vi "cic_interpolator_test_5_5cycles.vi"() -> ()   [LabVIEW 2013]
uses:
  <vilib>/measure/maspectr.llb/Power Spectrum and PSD Export Mode.ctl
  <vilib>/measure/maspectr.llb/FFT Power Spectrum and PSD for 1 Chan.vi
  <vilib>/measure/NI_MABase.lvlib
  <vilib>/measure/NI_MAPro.lvlib
panel:
  out "Waveform Graph out":dbl[](graph)
  out "Power spectrum in":cluster{"f0":dbl, "df":dbl, "magnitude":dbl[]}(graph)
  out "Power spectrum":cluster{"f0":dbl, "df":dbl, "magnitude":dbl[]}(graph)
  out "Waveform Graph":dbl[](graph)
  out "# of Iterations":i32
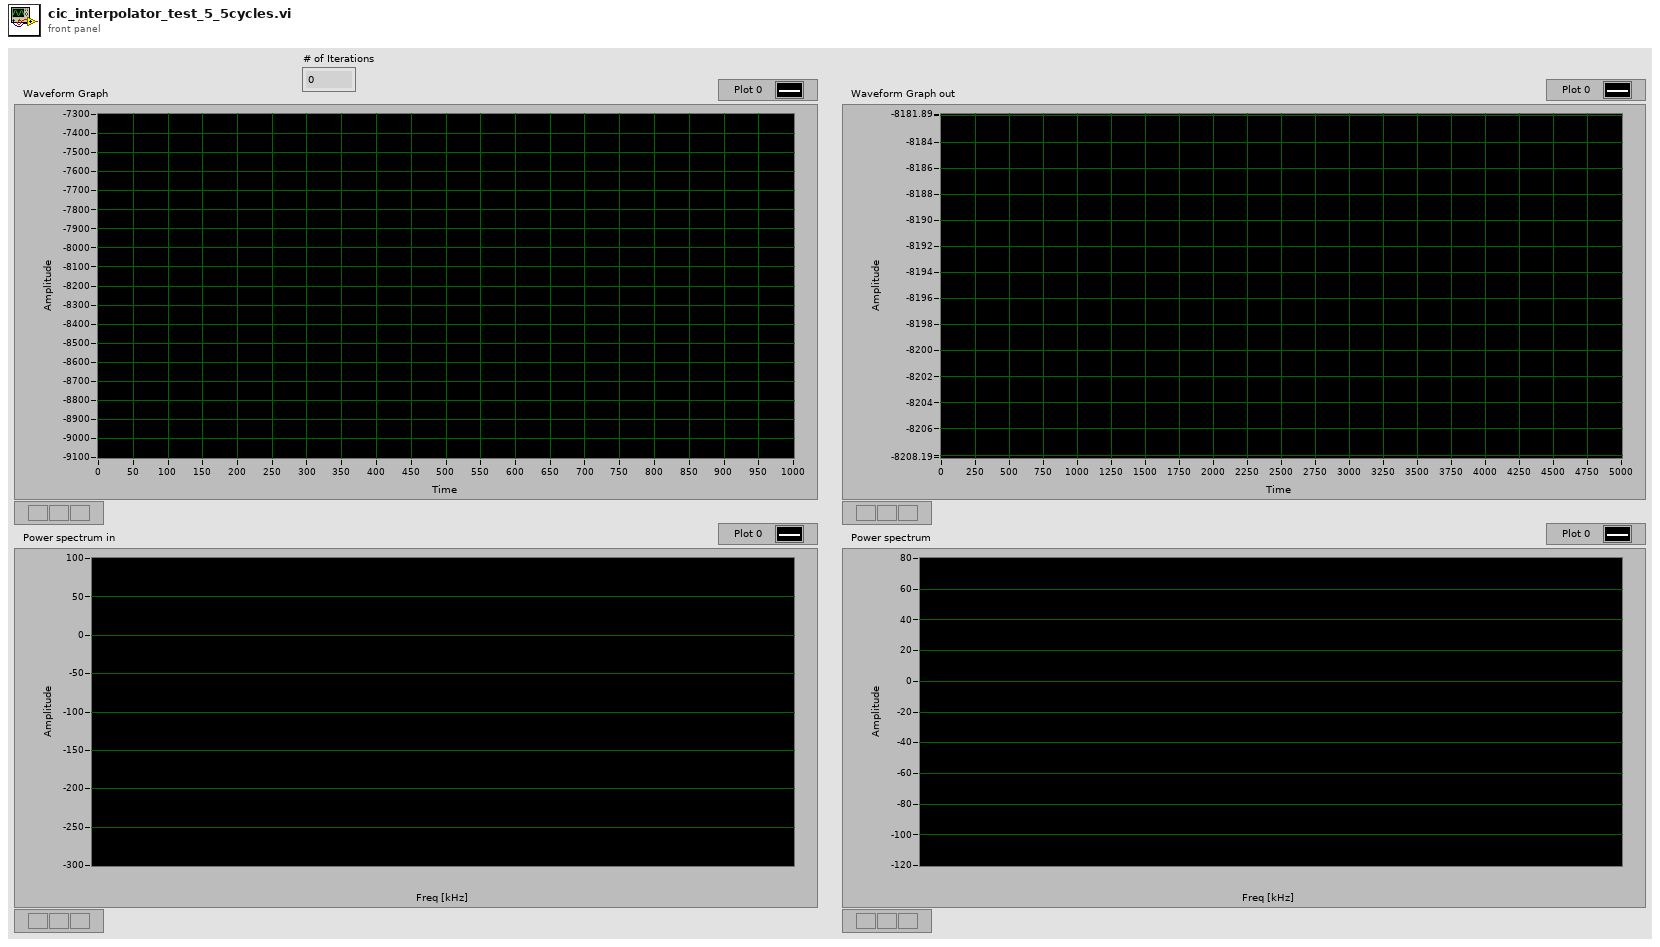
[diagram p1: front panel]
types:
  T1 = typedef "NI_MAPro.lvlib/Power Spectrum and PSD Export Mode.ctl" = u16
  T2 = cluster{"frequency":dbl, "amplitude":dbl, "phase":dbl}[]
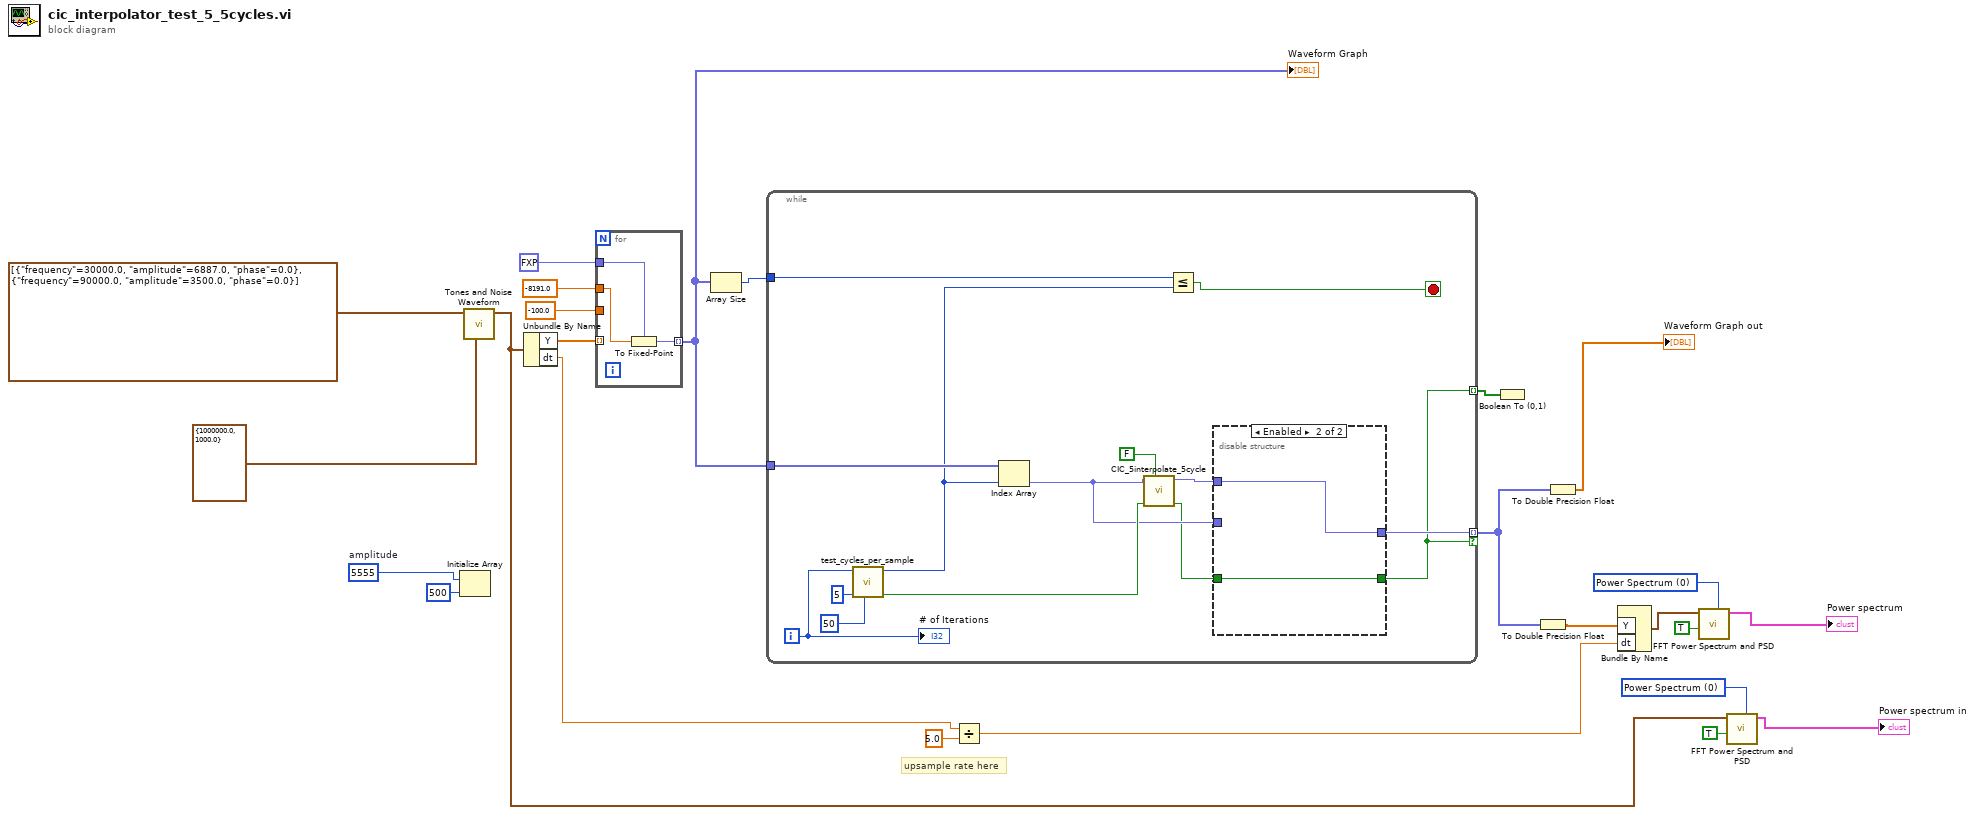
[diagram p0: block diagram]
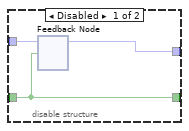
[diagram p2: hidden frame]
diagram:
  w4 = 5555  # amplitude
  w13 = T1 0 items=["Power Spectrum", "Power Spectral Density"] ("export mode")
  w21 = T1 0 items=["Power Spectrum", "Power Spectral Density"] ("export mode")
  # "upsample rate here"
  n1 = Initialize Array(w4, 500 ("dimension size")) -> ()  [unwired: 1 out]
  n2 = call <vilib>:"Tones and Noise Waveform.vi"("sampling info"=cluster{"Fs":dbl, "#s":dbl} {"Fs"=1000000.0, "#s"=1000.0}, "tones"=T2 [{"frequency"=30000.0, "amplitude"=6887.0, "phase"=0.0}, {"frequency"=90000.0, "amplitude"=3500.0, "phase"=0.0}]) -> ("signal out"=w12:waveform(dbl))  [unwired: 8 in, 1 out]
  n3 = Unbundle By Name(w12) -> ("Y"=w3:dbl[], "dt"=w19:dbl)
  n4 = for {
    tunnel: w3 -> [_] mode=indexing
    tunnel: fxp<+/-,16,14> 0.0 ("fixed-point type") -> [w28]
    tunnel: [w27] -> w6 mode=indexing
    tunnel: -8191.0 -> [w26]
    tunnel: -100.0 -> [_]
    n5 = To Fixed-Point(fixed-point type=w28, number=w26) -> (fixed-point=w27:fxp<+/-,16,14>)
  }
  "Waveform Graph" <- w6
  n6 = Array Size(array=w6) -> (size(s)=w7:i32)
  n7 = while {
    tunnel: w6 -> [w42]
    tunnel: [w31] -> w10 mode=indexing if=w29
    tunnel: w7 -> [w38]
    tunnel: [w29] -> w2 mode=indexing
    i -> [w41]
    stop <- w36 stop-if-true
    n8 = call "test_cycles_per_sample.vi"("initial delay"=50, "cycles per sample"=5, "index"=w41) -> ("valid out"=w34:bool, "array index"=w37:i32)  [unwired: 7 in]
    n9 = Index Array(array=w42, index=w37) -> (element=w33:fxp<+/-,16,14>)
    n10 = call "CIC_5interpolate_5cycle.vi"("reset"=FALSE, "valid in"=w34, "Data in"=w33) -> ("valid out"=w32:bool, "Data out"=w30:fxp<+/-,16,14>)  [unwired: 7 in]
    n11 = Less Or Equal?(x=w38, y=w37) -> (x <= y?=w36:bool)
    n12 = disable-structure shown="Enabled" {
      disable-tunnel: w33 -> [w45 _]
      disable-tunnel: w32 -> [w44 w46]
      disable-tunnel: [w44 w46] -> w29
      disable-tunnel: [w43 w47] -> w31
      disable-tunnel: w30 -> [_ w47]
      frame Disabled {
        n13 = feedback-in #1(w45, w44) -> ()
        n14 = feedback #1() -> (w43:fxp<+/-,16,14>)  [unwired: 1 in]
      }
      frame Enabled {
      }
    }
    "# of Iterations" <- w41
  }
  n15 = Divide(x=w19, y=5.0) -> (x/y=w17:dbl)
  n16 = Boolean To (0,1)(Boolean=w2) -> ()  [unwired: 1 out]
  n17 = To Double Precision Float(number=w10) -> (double precision float=w15:dbl[])
  n18 = To Double Precision Float(number=w10) -> (double precision float=→"Waveform Graph out":dbl[])
  n19 = Bundle By Name("Y"=w15, "dt"=w17) -> (w22:waveform(dbl))  [unwired: 1 in]
  n20 = call-poly <vilib>:"FFT Power Spectrum and PSD.vi"("export mode"=w21, "dB On (F)"=TRUE, "time signal"=w22) -> ("Power Spectrum / PSD"=→"Power spectrum":cluster{"f0":dbl, "df":dbl, "magnitude":dbl[]})  [unwired: 5 in, 3 out]
  n21 = call-poly <vilib>:"FFT Power Spectrum and PSD.vi"("export mode"=w13, "dB On (F)"=TRUE, "time signal"=w12) -> ("Power Spectrum / PSD"=→"Power spectrum in":cluster{"f0":dbl, "df":dbl, "magnitude":dbl[]})  [unwired: 5 in, 3 out]
